vi "Set Key.vi"(8 "error in (no error)":errorcluster, 9 "Define":bool=TRUE, 10 "Key":string, 11 "Stack in":T1[](array[typedef])) -> (0 "error out":errorcluster, 3 "Stack out":T1[](array[typedef]))   [LabVIEW 2015, in "TOML.lvlib"]
uses:
  TOML.lvlib
  Context.ctl
  Table Context.ctl
  Key-Value Pair.ctl
  Value.ctl
  Value Type.ctl
  Table Array Context.ctl
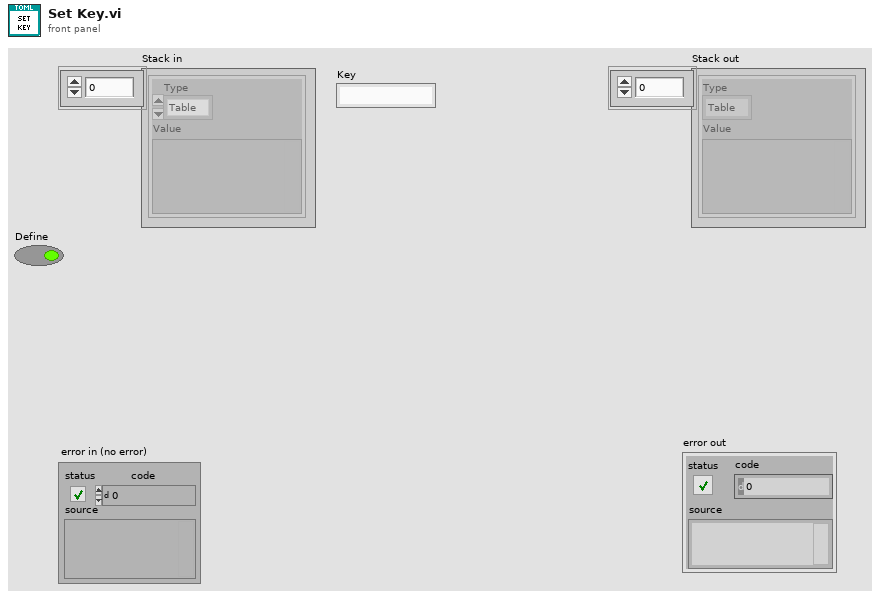
[diagram p1: front panel]
types:
  T1 = typedef "TOML.lvlib/Context.ctl" = cluster{"Type":enum16{"Table", "Array", "Inline Table", "Table Array"}, "Value":variant}
  T2 = typedef "TOML.lvlib/Table Context.ctl" = cluster{"Table":T3[], "Key":string, "Defined Keys":string[]}
  T3 = typedef "TOML.lvlib/Key-Value Pair.ctl" = cluster{"Key":string, "Value":T4}
  T4 = typedef "TOML.lvlib/Value.ctl" = cluster{"Type":T5, "Value":variant}
  T5 = typedef "TOML.lvlib/Value Type.ctl" = enum16{"Table", "Array", "String", "Integer", "Float", "Boolean", "Offset Date-Time", "Local Date-Time", "Local Date", "Local Time"}
  T6 = typedef "TOML.lvlib/Table Array Context.ctl" = cluster{"Table Array":cluster{"Table":T3[]}[], "Index":i32, "Key":string}
  T7 = enum16{"Table", "Array", "Inline Table", "Table Array"}
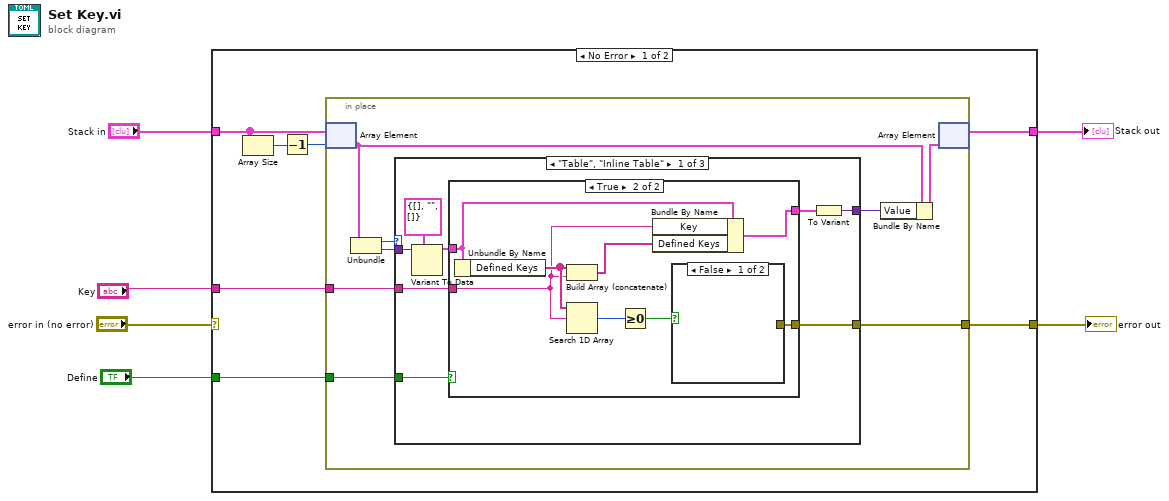
[diagram p0: block diagram]
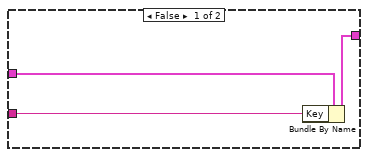
[diagram p2: hidden frame]
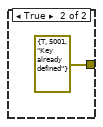
[diagram p3: hidden frame]
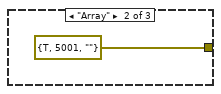
[diagram p4: hidden frame]
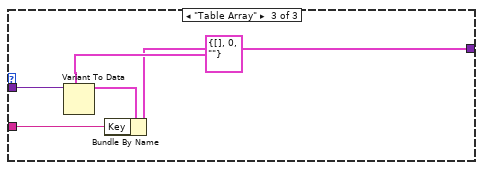
[diagram p5: hidden frame]
diagram:
  n1 = case shown="No Error" "error in (no error)" {
    selector: "error in (no error)" -> [_ w48]
    tunnel: "Stack in" -> [w11 w49]
    tunnel: [w10 w49] -> w5
    tunnel: "Key" -> [w9 _]
    tunnel: [w8 w48] -> w3
    tunnel: "Define" -> [w7 _]
    frame No Error {
      n2 = Array Size(array=w11) -> (size(s)=w13:i32)
      n3 = Decrement(x=w13) -> (x-1=w12:i32)
      n4 = in-place {
        in-place-border: w9 -> [w19]
        in-place-border: [w15] -> w8
        in-place-border: w7 -> [w14]
        n5 = in-place-array #1(w11, w12) -> (w18:T1)
        n6 = Unbundle(w18) -> ("Type"=w21:T7, "Value"=w20:variant)
        n7 = case shown="\"Table\", \"Inline Table\"" w21 {
          tunnel: w20 -> [w23 _ w47]
          tunnel: w19 -> [w29 _ w44]
          tunnel: [w27 _ w43] -> w17
          tunnel: [w22 errorcluster {"status"=TRUE, "code"=5001, "source"=""} ("error constant") _] -> w15
          tunnel: w14 -> [w26 _ _]
          frame "Table", "Inline Table" {
            n8 = Variant To Data(type=T2 {"Table"=[], "Key"="", "Defined Keys"=[]} ("Table Context"), Variant=w23) -> (data=w24:T2)  [unwired: 1 in, 1 out]
            n9 = case shown="True" w26 {
              tunnel: w29 -> [w32 w35]
              tunnel: [w31 w33] -> w28
              tunnel: w24 -> [w30 w36]
              tunnel: [_ w37] -> w22
              frame False {
                n10 = Bundle By Name(cluster=w30, "Key"=w32) -> (w31:T2)
              }
              frame True {
                n11 = Unbundle By Name(w36) -> ("Defined Keys"=w40:string[])
                n12 = Build Array (concatenate)(w40, w35) -> (w34:string[])
                n13 = Search 1D Array(1D array=w40, element=w35) -> (index of element=w39:i32)  [unwired: 1 in]
                n14 = Greater Or Equal To 0?(x=w39) -> (x >= 0?=w38:bool)
                n15 = Bundle By Name(cluster=w36, "Key"=w35, "Defined Keys"=w34) -> (w33:T2)
                n16 = case shown="False" w38 {
                  tunnel: [_ errorcluster {"status"=TRUE, "code"=5001, "source"="Key already defined"} ("error constant")] -> w37
                  frame False {
                  }
                  frame True {
                  }
                }
              }
            }
            n17 = To Variant(anything=w28) -> (Variant=w27:variant)
          }
          frame "Array" {
          }
          frame "Table Array" {
            n18 = Variant To Data(type=T6 {"Table Array"=[], "Index"=0, "Key"=""} ("Table Array Context"), Variant=w47) -> (data=w45:T6)  [unwired: 1 in, 1 out]
            n19 = Bundle By Name(cluster=w45, "Key"=w44) -> (w43:T6)
          }
        }
        n20 = Bundle By Name(cluster=w18, "Value"=w17) -> (w16:T1)
        n21 = in-place-array #1(w16) -> (w10:T1[])  [unwired: 1 out]
      }
    }
    frame Error {
    }
  }
  "Stack out" <- w5
  "error out" <- w3
